vi "Globals.vi"() -> ()   [LabVIEW 2015]
panel:
  in  "tester":dbl
  in  "Slider":dbl
  in  "VirtualSlider":dbl
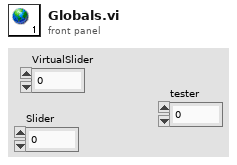
[diagram p1: front panel]
diagram:
